vi "ExponentialMovingAverage.vi"(2 "old value":dbl=0.51444, 3 "current value":dbl=0.51444, 4 "weight":dbl=0.51444) -> (1 "average":dbl=0.51444)   [LabVIEW 2013]
doc: "Takes a new value, an old value, and the weight that should be given to the old value when averaging, and returns a weighted average."
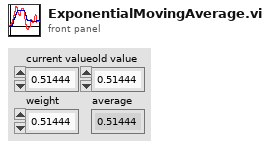
[diagram p1: front panel]
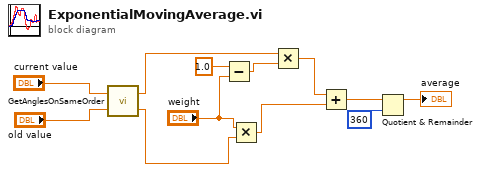
[diagram p0: block diagram]
diagram:
  n1 = call "GetAnglesOnSameOrder.vi"("Angle 2"="old value", "Angle 1"="current value") -> ("Wrapped A2"=w4:dbl, "Wrapped A1"=w6:dbl)
  n2 = Subtract(x=1.0, y="weight") -> (x-y=w10:dbl)
  n3 = Multiply(x="weight", y=w4) -> (x*y=w8:dbl)
  n4 = Multiply(x=w6, y=w10) -> (x*y=w9:dbl)
  n5 = Add(x=w9, y=w8) -> (x+y=w1:dbl)
  n6 = Quotient & Remainder(x=w1, y=360) -> (x-y*floor(x/y)=→"average":dbl)  [unwired: 1 out]
